vi "Draw Elements On Field.vi"(1 "CoordinatesArray [x, y, intensity]":cluster{"X":dbl, "Y":dbl, "Intensity":dbl}[](array[cluster]), 2 "Field In":dbl[][](graph)) -> (0 "Field Out":dbl[][](graph))   [LabVIEW 2014, in "Field.lvclass"]
uses:
  Field.lvclass
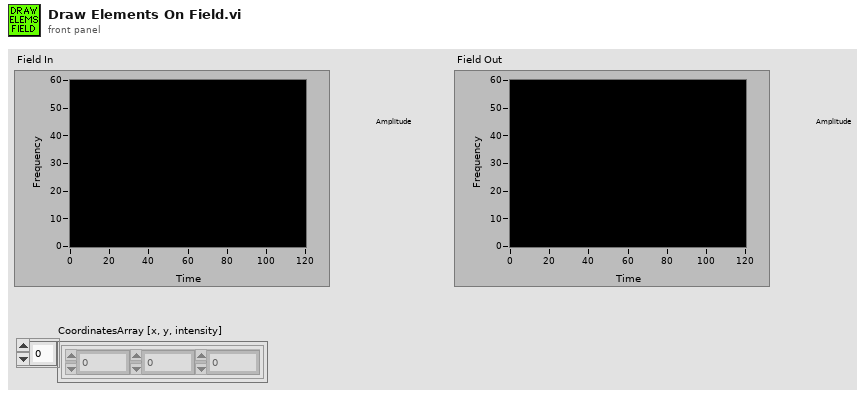
[diagram p1: front panel]
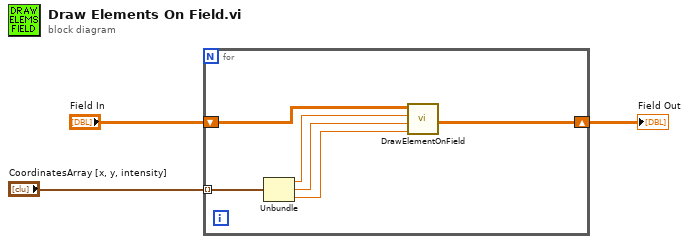
[diagram p0: block diagram]
diagram:
  n1 = for {
    tunnel: "CoordinatesArray [x, y, intensity]" -> [w9] mode=indexing
    shift-right: [w4] -> w1
    shift-left: "Field In" -> [w5]
    n2 = Unbundle(w9) -> ("X"=w8:dbl, "Y"=w7:dbl, "Intensity"=w6:dbl)
    n3 = call "DrawElementOnField.vi"("Intensity"=w6, "PosY"=w7, "PosX"=w8, "Field in"=w5) -> ("Field out"=w4:dbl[][])
  }
  "Field Out" <- w1
